vi "Controller Data Server Loop.vi"(4 "Log File Reference":refnum<file>, 7 "Sync Objects":T1, 8 "error in (no error)":errorcluster, 11 "FOFB Configuration":T5={"FOFB Parameters"={"Network"={"FOFB Controller IP"="", "LNLS Control Network IP"="", "LNLS Control Network Power Supplies TCP Port"=0, "LNLS Control Network FOFB Configuration TCP Port"=0, "Data Server TCP Port"=0, "Monitoring Data TCP Port"=0, "Configuration GUI TCP Port"=0, "TCP Listening Timeout"=0}, "Fast Acquisition"={"Acquisition Period"=0, "Data Buffer Size"=0, "Monitoring Period"=0}, "Response Matrix Measurement"={"Step Amplitude"=0.0, "Time Between Steps"=0, "Step Duration"=0, "Number of Averages"=0}, "Correction Algorithm"={"Correction Period"=0, "Reference Orbit Path"=path "", "Response Matrix Path"=path "", "Correction Matrix Path"=path "", "Horizontal Correction Factor"=0.0, "Vertical Correction Factor"=0.0, "Beam Current FOFB Threshold"=0.0, "Decouple H-V"=FALSE, "Use Additional BPM LPF"=FALSE, "BPM LPF Cutoff"=0.0}, "Acquisition Network"=[], "Actuation Network"=[]}, "Number of Acquisition Chassis"=0, "Number of Actuation Chassis"=0, "Number of BPM Readings"=0, "BPM Reading Names"=[], "Selected BPM Readings"=[0, 1, 2, 3, 4, 5, 6, 7, 8, 9, 10, 11, 12, 13, 14, 15, 16, 17, 18, 19, 20, 21, 22, 23, 24, 25, 26, 27, 28, 29, 30, 31, 32, 33, 34, 35, 36, 37, 38, 39, 40, 41, 42, 43, 44, 45, 46, 47, 48, 49], "Number of Correctors"=0, "Corrector Names"=[], "Selected Correctors"=[0, 1, 2, 3, 4, 5, 6, 7, 8, 9, 10, 11, 12, 13, 14, 15, 16, 17, 18, 19, 20, 21, 22, 23, 24, 25, 26, 27, 28, 29, 30, 31, 32, 33, 34, 35, 36, 37, 38, 39, 40, 41, 42, 43, 44, 45, 46, 47, 48, 49], "Reference Orbit"=[], "Response Matrix"=[], "Correction Matrix"=[], "Acquisition Chassis Names"=[], "Actuation Chassis Names"=[], "Acquisition Variables"=[], "Actuation Variables"=[], "PS Matrix Mapping"=[], "Inverse PS Matrix Mapping"=[], "Response Matrix Beam Energy (MeV)"=0.0, "PID Parameters"=[], "BPM Planes"=[], "Corrector Planes"=[], "RMM Step Factor"=[]}) -> (0 "error out":errorcluster)   [LabVIEW 2011, in "Controller VIs.lvlib"]
uses:
  Controller VIs.lvlib
  Types Definitions/Type FOFB Configuration.ctl
  Types Definitions/Type FOFB Parameters.ctl
  Types Definitions/Type Network Configuration.ctl
  Types Definitions/Type FA Configuration.ctl
  Types Definitions/Type Response Matrix Measurement Configuration.ctl
  Types Definitions/Type Correction Algorithm Configuration.ctl
  Types Definitions/Type Acquisition Network Configuration.ctl
  Types Definitions/Type Actuation Network Configuration.ctl
  Types Definitions/Type PID Parameters.ctl
  Types Definitions/Type Synchronization Objects.ctl
  Types Definitions/Type Blocking Synchronization Objects.ctl
  Types Definitions/Type FA Request Parameters.ctl
  Types Definitions/Type BPM and PS select cluster.ctl
  Types Definitions/Type FA File Parameters.ctl
  Types Definitions/Type Monitoring Data.ctl
  Types Definitions/Type Diagnostics Data.ctl
  Types Definitions/Type CPU Loads Array.ctl
  Types Definitions/Type CPU Loads.ctl
  Types Definitions/Type Non-blocking Synchronization Objects.ctl
  Types Definitions/Type FOFB Variables.ctl
  Types Definitions/Type Actuation State.ctl
  <vilib>/Platform/TimedLoop/XDataNode/timing_clust.ctl
  <vilib>/Platform/TimedLoop/XDataNode/nitl_modes.ctl
  <vilib>/Platform/TimedLoop/XDataNode/wakeup.ctl
  <vilib>/rtutility.llb/RT Debug String.vi
  <vilib>/Platform/TimedLoop/XDataNode/XDataNode.xnode
  Data Server VIs.lvlib
  Log VIs.lvlib
  Type Definitions.lvlib
  <vilib>/Platform/TimedLoop/XDataNode/XDNodeRunTimeDep.lvlib
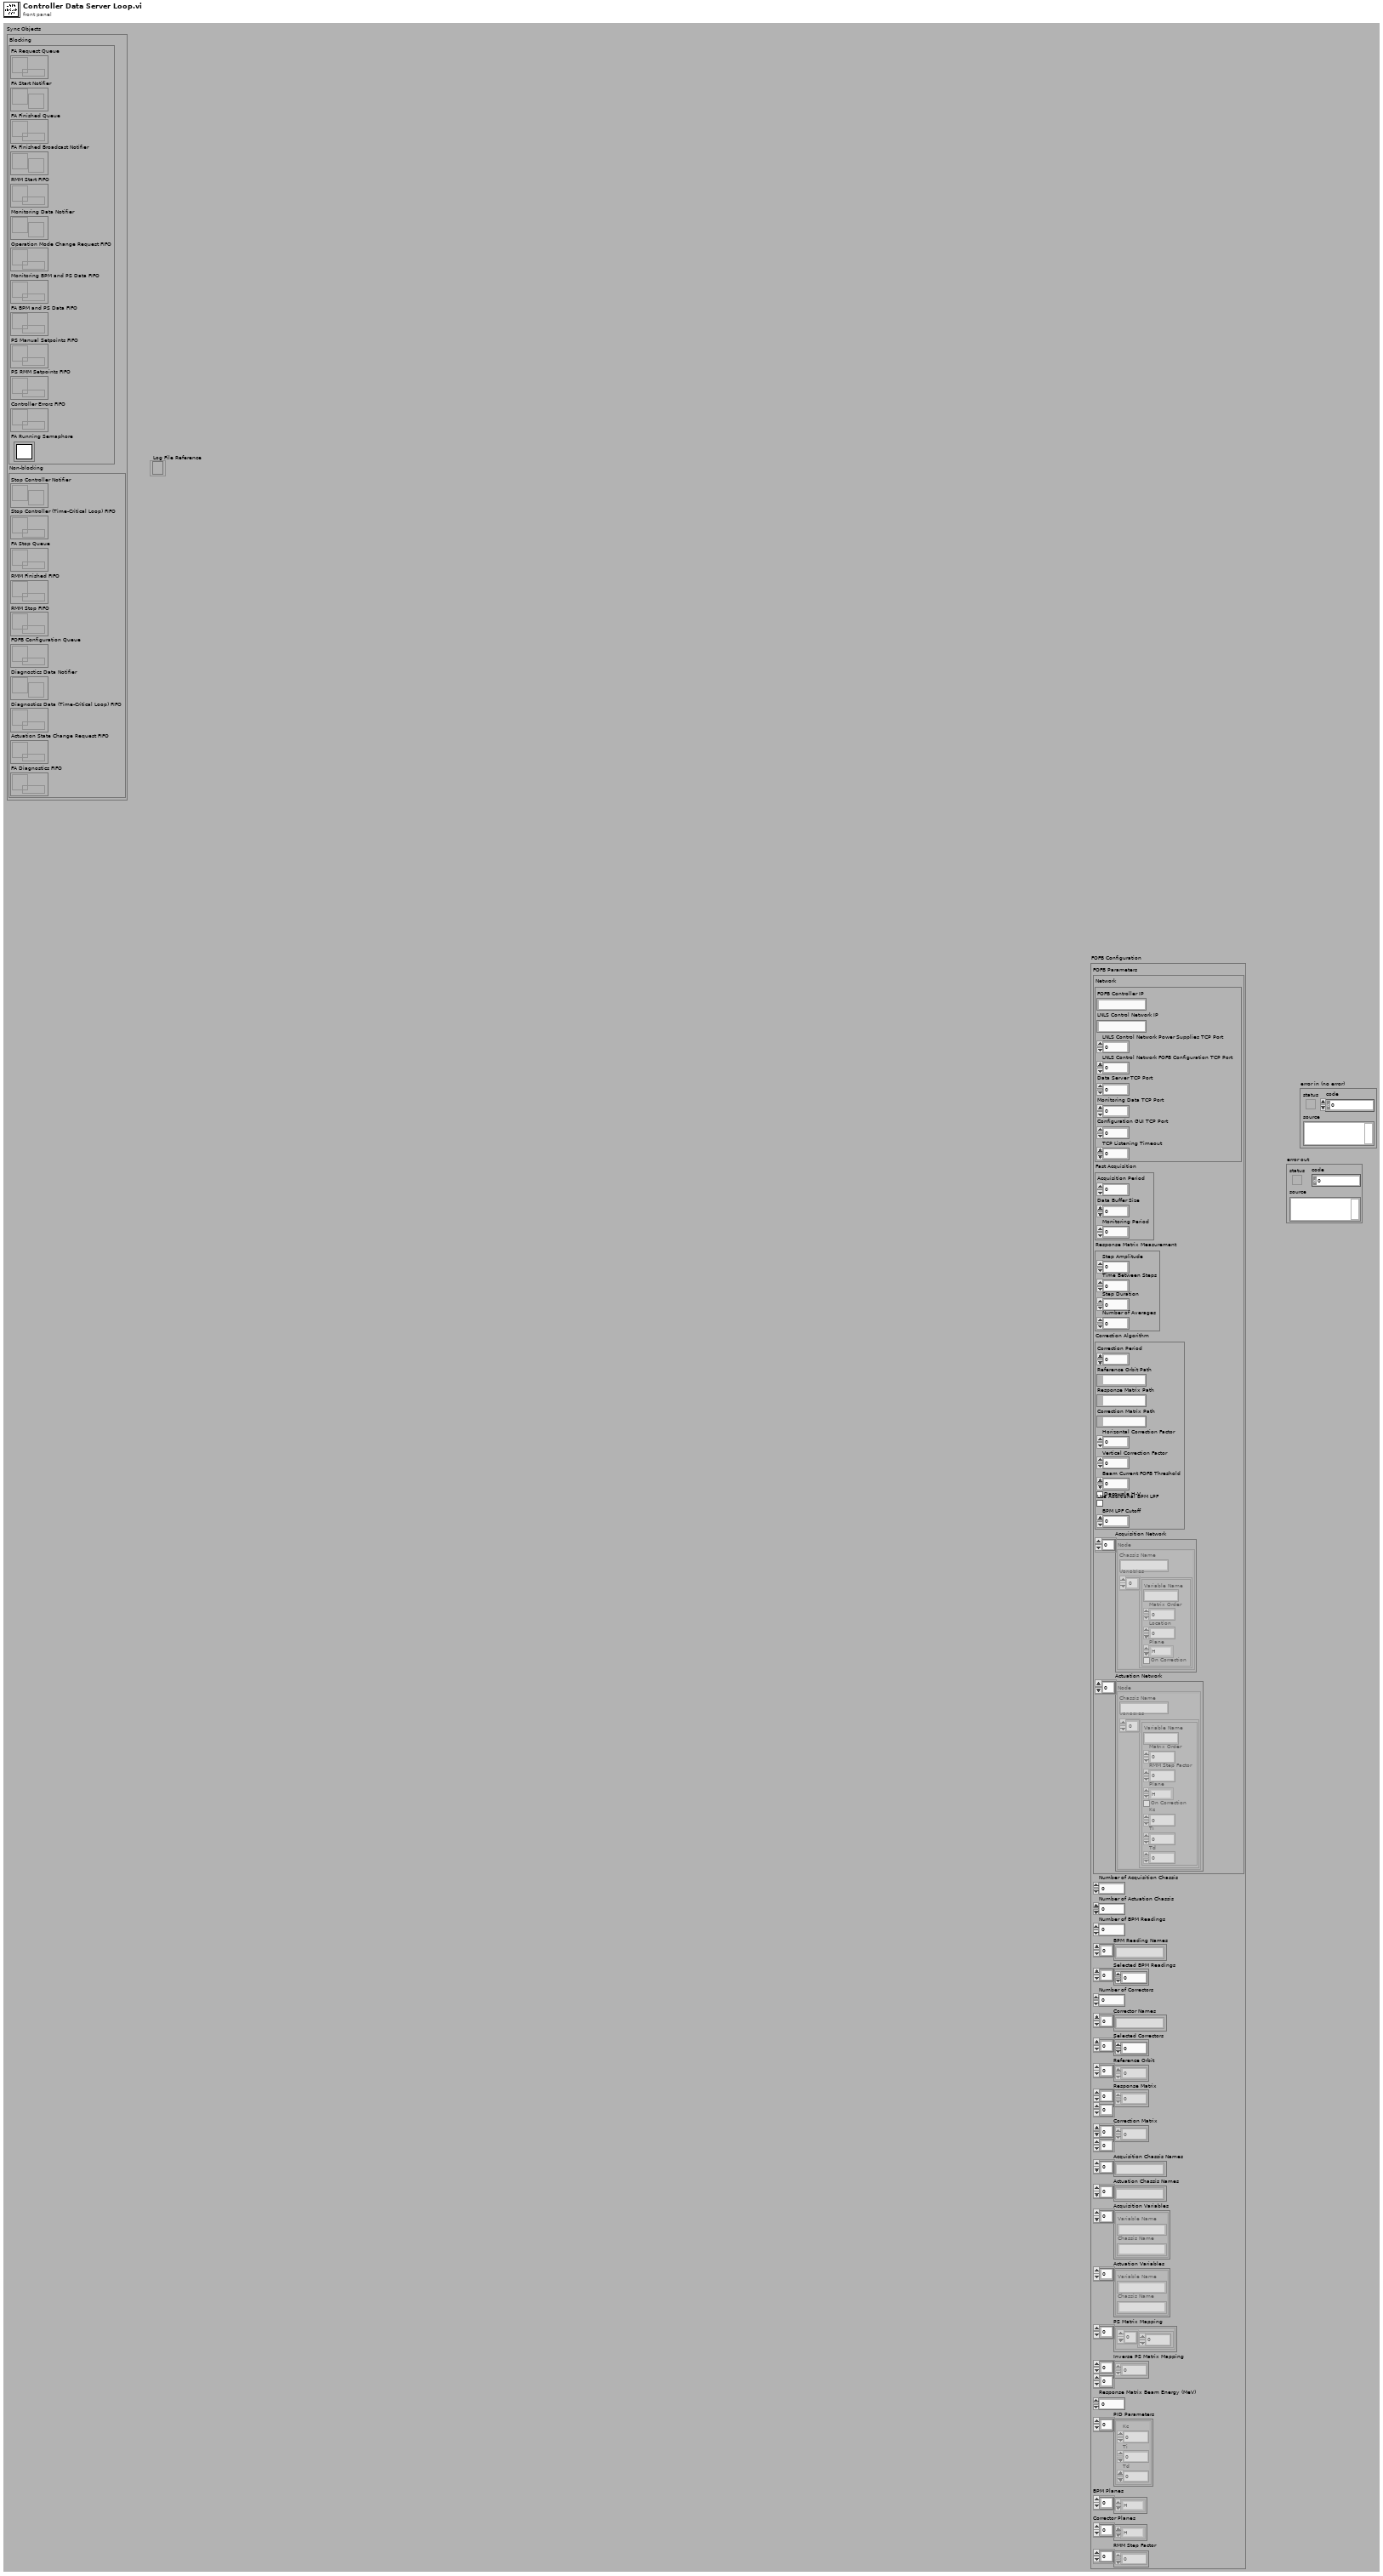
[diagram p1: front panel]
types:
  T1 = typedef "Type Definitions.lvlib/Type Synchronization Objects.ctl" = cluster{"Blocking":T2, "Non-blocking":T4}
  T2 = typedef "Type Definitions.lvlib/Type Blocking Synchronization Objects.ctl" = cluster{"FA Request Queue":refnum<queue>, "FA Start Notifier":refnum<notifier>, "FA Finished Queue":refnum<queue>, "FA Finished Broadcast Notifier":refnum<notifier>, "RMM Start FIFO":refnum<k33>, "Monitoring Data Notifier":refnum<notifier>, "Operation Mode Change Request FIFO":refnum<k33>, "Monitoring BPM and PS Data FIFO":refnum<k33>, "FA BPM and PS Data FIFO":refnum<k33>, "PS Manual Setpoints FIFO":refnum<k33>, "PS RMM Setpoints FIFO":refnum<k33>, "Controller Errors FIFO":refnum<k33>, "FA Running Semaphore":T3}
  T3 = typedef "Semaphore RefNum" = refnum<k1>
  T4 = typedef "Type Definitions.lvlib/Type Non-blocking Synchronization Objects.ctl" = cluster{"Stop Controller Notifier":refnum<notifier>, "Stop Controller (Time-Critical Loop) FIFO":refnum<k33>, "FA Stop Queue":refnum<queue>, "RMM Finished FIFO":refnum<k33>, "RMM Stop FIFO":refnum<k33>, "FOFB Configuration Queue":refnum<queue>, "Diagnostics Data Notifier":refnum<notifier>, "Diagnostics Data (Time-Critical Loop) FIFO":refnum<k33>, "Actuation State Change Request FIFO":refnum<k33>, "FA Diagnostics FIFO":refnum<k33>}
  T5 = typedef "Type Definitions.lvlib/Type FOFB Configuration.ctl" = cluster{"FOFB Parameters":T6, "Number of Acquisition Chassis":i32, "Number of Actuation Chassis":i32, "Number of BPM Readings":i32, "BPM Reading Names":string[], "Selected BPM Readings":u32[], "Number of Correctors":i32, "Corrector Names":string[], "Selected Correctors":u32[], "Reference Orbit":dbl[], "Response Matrix":dbl[][], "Correction Matrix":dbl[][], "Acquisition Chassis Names":string[], "Actuation Chassis Names":string[], "Acquisition Variables":cluster{"Variable Name":string, "Chassis Name":string}[], "Actuation Variables":cluster{"Variable Name":string, "Chassis Name":string}[], "PS Matrix Mapping":cluster{u32[]}[], "Inverse PS Matrix Mapping":u32[][], "Response Matrix Beam Energy (MeV)":dbl, "PID Parameters":T13[], "BPM Planes":enum8{"H", "V"}[], "Corrector Planes":enum8{"H", "V"}[], "RMM Step Factor":dbl[]}
  T6 = typedef "Type Definitions.lvlib/Type FOFB Parameters.ctl" = cluster{"Network":T7, "Fast Acquisition":T8, "Response Matrix Measurement":T9, "Correction Algorithm":T10, "Acquisition Network":T11, "Actuation Network":T12}
  T7 = typedef "Type Definitions.lvlib/Type Network Configuration.ctl" = cluster{"FOFB Controller IP":string, "LNLS Control Network IP":string, "LNLS Control Network Power Supplies TCP Port":u16, "LNLS Control Network FOFB Configuration TCP Port":u16, "Data Server TCP Port":u16, "Monitoring Data TCP Port":u16, "Configuration GUI TCP Port":u16, "TCP Listening Timeout":i32}
  T8 = typedef "Type Definitions.lvlib/Type FA Configuration.ctl" = cluster{"Acquisition Period":u32, "Data Buffer Size":u32, "Monitoring Period":u32}
  T9 = typedef "Type Definitions.lvlib/Type Response Matrix Measurement Configuration.ctl" = cluster{"Step Amplitude":dbl, "Time Between Steps":u32, "Step Duration":u32, "Number of Averages":u32}
  T10 = typedef "Type Definitions.lvlib/Type Correction Algorithm Configuration.ctl" = cluster{"Correction Period":u32, "Reference Orbit Path":path, "Response Matrix Path":path, "Correction Matrix Path":path, "Horizontal Correction Factor":dbl, "Vertical Correction Factor":dbl, "Beam Current FOFB Threshold":dbl, "Decouple H-V":bool, "Use Additional BPM LPF":bool, "BPM LPF Cutoff":dbl}
  T11 = typedef "Type Definitions.lvlib/Type Acquisition Network Configuration.ctl" = cluster{"Chassis Name":string, "Variables":cluster{"Variable Name":string, "Matrix Order":u32, "Location":dbl, "Plane":enum8{"H", "V"}, "On Correction":bool}[]}[]
  T12 = typedef "Type Definitions.lvlib/Type Actuation Network Configuration.ctl" = cluster{"Chassis Name":string, "Variables":cluster{"Variable Name":string, "Matrix Order":u32, "RMM Step Factor":dbl, "Plane":enum8{"H", "V"}, "On Correction":bool, "Kc":dbl, "Ti":dbl, "Td":dbl}[]}[]
  T13 = typedef "Type Definitions.lvlib/Type PID Parameters.ctl" = cluster{"Kc":fxp<+/-,16,8>, "Ti":fxp<+/-,16,8>, "Td":fxp<+/-,16,8>}
  T14 = enum16{"Wait Connection", "Read Data 1", "Write Data", "Read Data 2", "Close Connection", "Idle"}
  T15 = typedef "XDNodeRunTimeDep.lvlib/timing_clust.ctl" = cluster{"Expected End [f-1]":u64, "Actual End [f-1]":u64, "Finished Late? [f-1]":bool, "Expected End [i-1]":u64, "Actual End [i-1]":u64, "Finished Late? [i-1]":bool, "Expected Start [i]":u64, "Actual Start [i]":u64, "Expected Start [f]":u64, "Actual Start [f]":u64, "Source Name":string, "Structure Name":string, "Period":i64, "Deadline":i64, "Offset":i64, "Start":i64, "Priority":i32, "Timeout":i32, "Mode":T16, "Wakeup Reason":T17, "Error":errorcluster, "Source Type":string, "Secondary Source Type":string, "Global End Time":u64, "Global Start Time":u64, "Frame Duration":u64, "Iteration Duration":u64, "Assigned CPU":i32, "I/O Scan Engine Mode":u32}
  T16 = typedef "XDNodeRunTimeDep.lvlib/nitl_modes.ctl" = enum32{"No Change", "Process missed periods, maintain original phase", "Discard missed periods, maintain original phase", "Process missed periods, ignore original phase", "Discard missed periods, ignore original phase"}
  T17 = typedef "XDNodeRunTimeDep.lvlib/wakeup.ctl" = enum32{"Normal", "Aborted", "Asynchronous wakeup", "Timing source error", "Timed loop error", "Timeout"}
  T18 = enum16{"Standard", "Buffered", "CRLF", "Immediate"}
  T19 = typedef "Type Definitions.lvlib/Type FA Request Parameters.ctl" = cluster{"Number of Samples":u32, "BPM and PS Selection":T20, "Filename":string}
  T20 = typedef "Type Definitions.lvlib/Type BPM and PS select cluster.ctl" = cluster{"BPM index array":u32[], "PS index array ":u32[]}
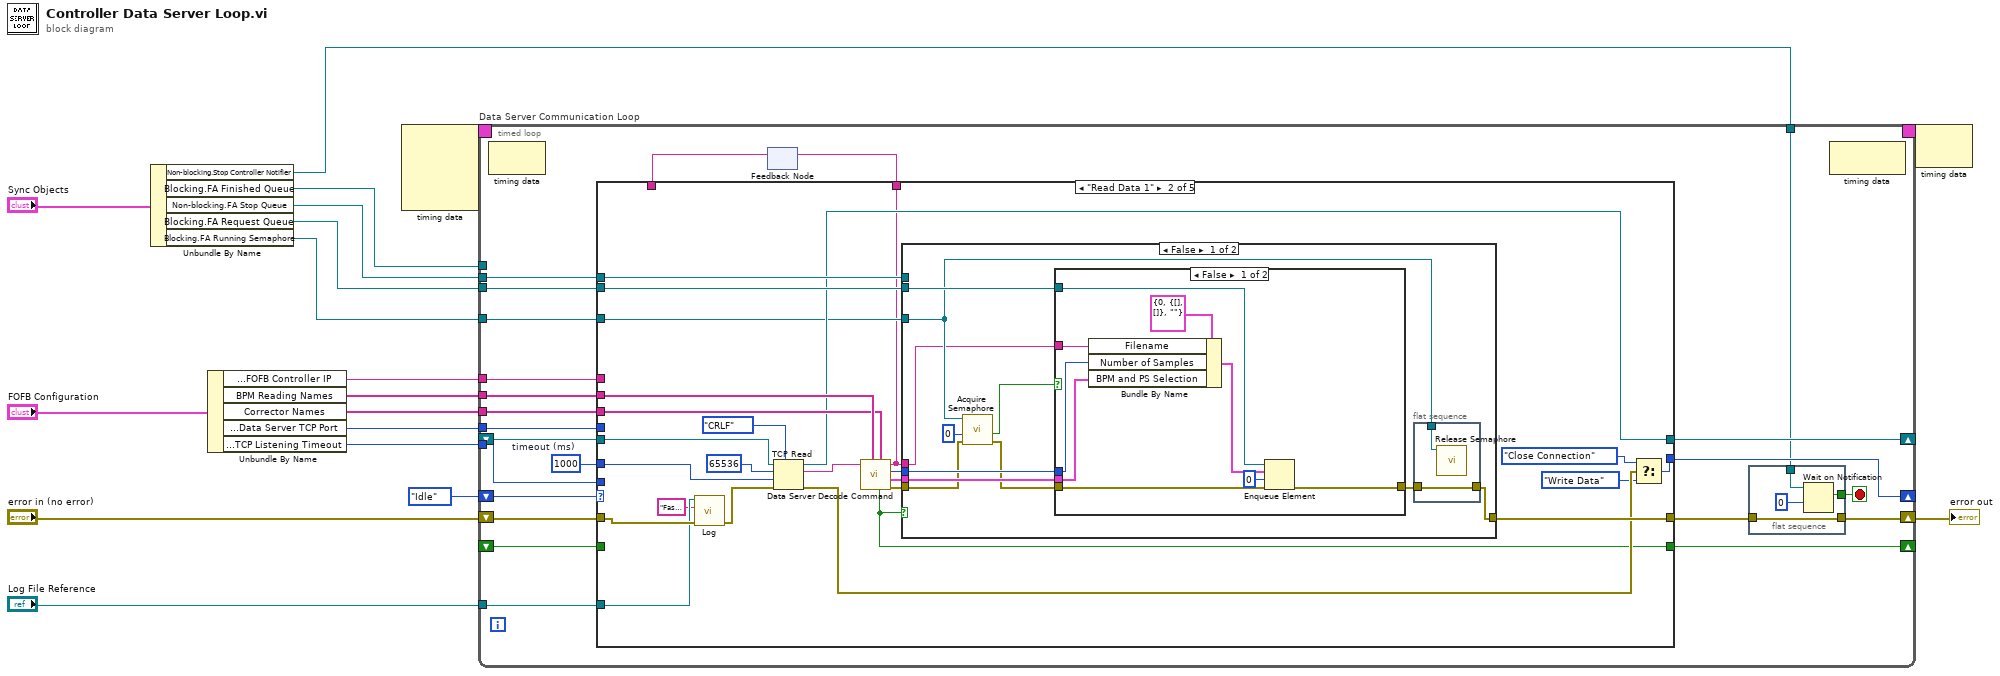
[diagram p0: block diagram]
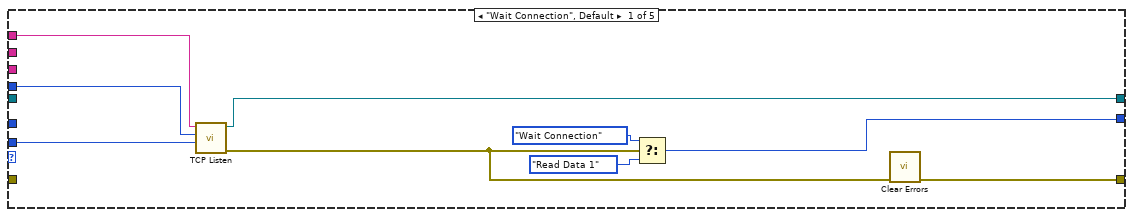
[diagram p2: hidden frame]
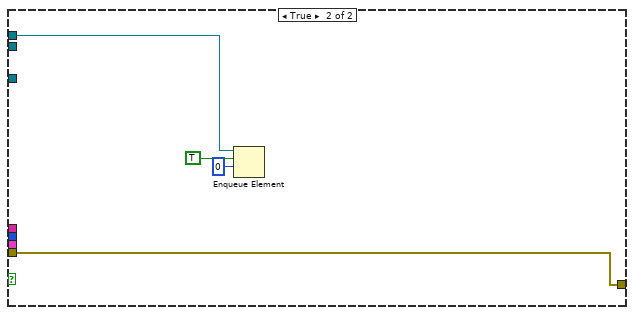
[diagram p4: hidden frame]
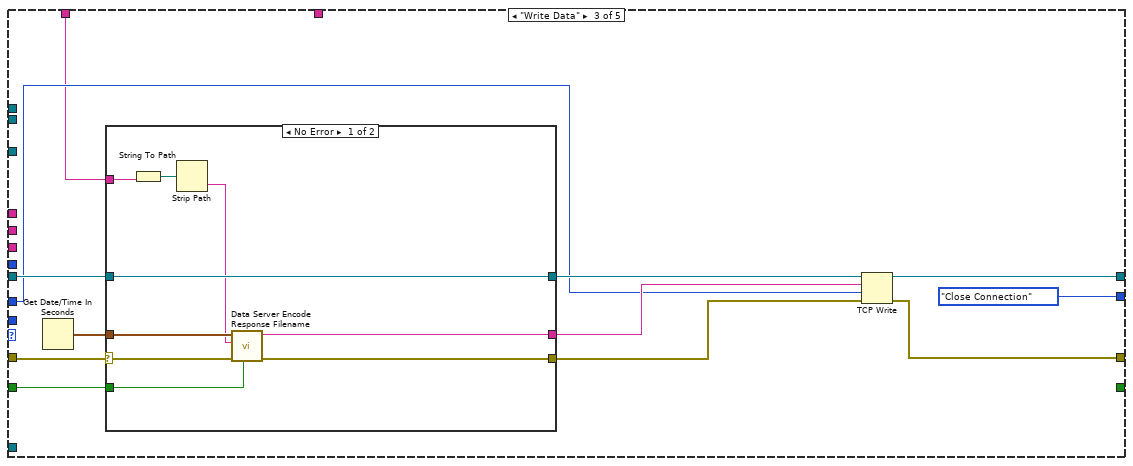
[diagram p5: hidden frame]
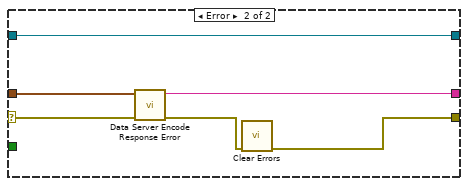
[diagram p6: hidden frame]
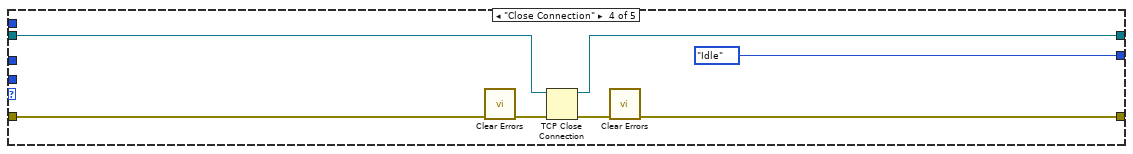
[diagram p7: hidden frame]
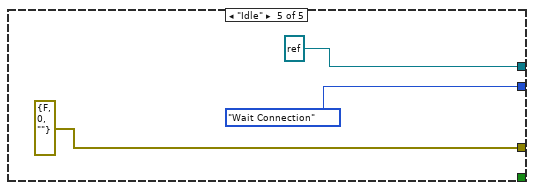
[diagram p8: hidden frame]
diagram:
  n1 = Unbundle By Name("Sync Objects") -> ("Non-blocking.Stop Controller Notifier"=w8:refnum<notifier>, "Blocking.FA Finished Queue"=w4:refnum<queue>, "Non-blocking.FA Stop Queue"=w6:refnum<queue>, "Blocking.FA Request Queue"=w7:refnum<queue>, "Blocking.FA Running Semaphore"=w3:T3)
  n2 = Unbundle By Name("FOFB Configuration") -> ("FOFB Parameters.Network.FOFB Controller IP"=w11:string, "BPM Reading Names"=w12:string[], "Corrector Names"=w13:string[], "FOFB Parameters.Network.Data Server TCP Port"=w9:u16, "FOFB Parameters.Network.TCP Listening Timeout"=w5:i32)
  n3 = node-c288() -> (w2:T15)  [unwired: 4 in]
  n4 = timed-loop "Data Server Communication Loop" {
    shift-right: [w40] -> _
    shift-left: _ -> [w37]
    shift-right: [w39] -> _
    shift-left: T14."Idle" ("f") -> [w41]
    shift-right: [w27] -> w15
    shift-left: "error in (no error)" -> [w38]
    tunnel: w12 -> [w35]
    tunnel: w13 -> [w34]
    tunnel: w11 -> [w33]
    tunnel: w9 -> [w31]
    tunnel: w8 -> [w30]
    tunnel: "Log File Reference" -> [w29]
    tunnel: w7 -> [w26]
    tunnel: w6 -> [w25]
    tunnel: w5 -> [w24]
    shift-right: [w23] -> _
    shift-left: _ -> [w22]
    tunnel: w4 -> [_]
    tunnel: w3 -> [w21]
    timing: w2 -> [_]
    timing-out: [_] -> w1
    stop <- w32 stop-if-true
    w36 = 1000  # timeout (ms)
    # "ms"
    n5 = node-c288() -> ()  [unwired: 1 in, 1 out]
    n6 = feedback #1() -> (w20:string)  [unwired: 1 in]
    n7 = case shown="\"Read Data 1\"" w41 {
      tunnel: [w56 w59 w115 w140 refnum<k5> refnum ("connection ID")] -> w40
      tunnel: [w53 w65 T14."Close Connection" ("f") T14."Idle" ("f") T14."Wait Connection" ("f")] -> w39
      tunnel: [w49 w66 w111 w139 errorcluster {"status"=FALSE, "code"=0, "source"=""} ("error out")] -> w28
      tunnel: w38 -> [_ w74 w120 w136 _]
      tunnel: w37 -> [_ w79 w118 w141 _]
      tunnel: w36 -> [_ w78 w113 _ _]
      tunnel: w35 -> [_ w76 _ _ _]
      tunnel: w34 -> [_ w75 _ _ _]
      tunnel: w33 -> [w52 _ _ _ _]
      tunnel: w31 -> [w51 _ _ _ _]
      tunnel: w29 -> [_ w72 _ _ _]
      tunnel: w26 -> [_ w70 _ _ _]
      tunnel: w25 -> [_ w61 _ _ _]
      tunnel: w24 -> [w48 _ _ _ _]
      tunnel: w22 -> [_ _ w110 _ _]
      tunnel: [_ w60 _ _ _] -> w23
      tunnel: w21 -> [_ w58 _ _ _]
      tunnel: w20 -> [_ _ w109 _ _]
      tunnel: [_ w57 _ _ _] -> w19
      frame "Wait Connection", Default {
        n8 = call <vilib>:"TCP Listen.vi"("timeout ms (wait forever: -1)"=w48, "port"=w51, "service name"=w52) -> ("error out"=w50:errorcluster, "connection ID"=w56:refnum<k5>)  [unwired: 4 in, 3 out]
        n9 = Select(t=T14."Wait Connection" ("f"), s=w50, f=T14."Read Data 1") -> (s? t:f=w53:T14)
        n10 = call <vilib>:"Clear Errors.vi"("error in (no error)"=w50) -> ("error out"=w49:errorcluster)  [unwired: 6 out]
      }
      frame "Read Data 1" {
        n11 = call "Log.vi"("error in (no error)"=w74, "String"="Fast Acquisition requested by user.", "Log File Reference"=w72) -> ("error out"=w73:errorcluster)  [unwired: 7 in, 1 out]
        n12 = TCP Read(connection ID=w79, bytes to read=65536, error in (no error)=w73, 7:T18."CRLF" ("mode (standard)"), 9:w78) -> (connection ID out=w59:refnum<k5>, data out=w77:string, error out=w63:errorcluster)
        n13 = call "Data Server Decode Command.vi"("Corrector names"=w75, "BPM names"=w76, "Input string"=w77) -> ("error out"=w67:errorcluster, "BPM and PS index"=w68:T20, "Number of samples"=w69:u32, "Filename"=w57:string, "Stop Acquisition?"=w60:bool)  [unwired: 4 in]
        n14 = case shown="False" w60 {
          tunnel: w70 -> [w92 _]
          tunnel: w69 -> [w91 _]
          tunnel: w68 -> [w90 _]
          tunnel: w67 -> [w88 w108]
          tunnel: [w83 w108] -> w66
          tunnel: w61 -> [_ w107]
          tunnel: w58 -> [w85 _]
          tunnel: w57 -> [w82 _]
          frame False {
            n15 = call <vilib>:"Acquire Semaphore.vi"("error in (no error)"=w88, "ms timeout (-1)"=0, "semaphore"=w85) -> ("error out"=w87:errorcluster, "timed out"=w86:bool)  [unwired: 2 in, 1 out]
            n16 = case shown="False" w86 {
              tunnel: w92 -> [w99 _]
              tunnel: w91 -> [w102 _]
              tunnel: w90 -> [w101 _]
              tunnel: w82 -> [w100 _]
              tunnel: [w95 w104] -> w84
              tunnel: w87 -> [w97 w104]
              frame False {
                n17 = Bundle By Name(cluster=T19 {"Number of Samples"=0, "BPM and PS Selection"={"BPM index array"=[], "PS index array "=[]}, "Filename"=""} ("notification"), "Filename"=w100, "Number of Samples"=w102, "BPM and PS Selection"=w101) -> (w98:T19)
                n18 = Enqueue Element(queue=w99, element=w98, timeout in ms (-1)=0, error in (no error)=w97) -> (error out=w95:errorcluster)  [unwired: 2 out]
              }
              frame True {
              }
            }
            n19 = flat-sequence {
              tunnel: w85 -> [w94]
              tunnel: w84 -> [w93]
              tunnel: [w93] -> w83
              frame #0 {
                n20 = call <vilib>:"Release Semaphore.vi"("semaphore"=w94) -> ()  [unwired: 5 in, 2 out]
              }
            }
          }
          frame True {
            n21 = Enqueue Element(queue=w107, element=TRUE ("notification"), timeout in ms (-1)=0) -> ()  [unwired: 1 in, 3 out]
          }
        }
        n22 = Select(t=T14."Close Connection" ("f"), s=w63, f=T14."Write Data") -> (s? t:f=w65:T14)
      }
      frame "Write Data" {
        n23 = Get Date/Time In Seconds() -> (seconds since 1Jan1904=w119:timestamp)
        n24 = case shown="No Error" w120 {
          selector: w120 -> [w128 w135]
          tunnel: w119 -> [w129 w134]
          tunnel: [w125 w130] -> w116
          tunnel: w118 -> [w127 w133]
          tunnel: [w127 w133] -> w117
          tunnel: [w126 w131] -> w114
          tunnel: w109 -> [w124 _]
          tunnel: w110 -> [w121 _]
          frame No Error {
            n25 = String To Path(string=w124) -> (path=w123:path)
            n26 = Strip Path(path=w123) -> (name=w122:string)  [unwired: 1 out]
            n27 = call "Data Server Encode Response Filename.vi"("FA Stopped?"=w121, "error in (no error)"=w128, "Filename"=w122, "Time Stamp"=w129) -> ("error out"=w126:errorcluster, "Output string"=w125:string)  [unwired: 6 in]
          }
          frame Error {
            n28 = call "Data Server Encode Response Error.vi"("error in (no error)"=w135, "Time Stamp"=w134) -> ("error out"=w132:errorcluster, "Output string"=w130:string)  [unwired: 8 in]
            n29 = call <vilib>:"Clear Errors.vi"("error in (no error)"=w132) -> ("error out"=w131:errorcluster)  [unwired: 6 in]
          }
        }
        n30 = TCP Write(connection ID=w117, data in=w116, error in (no error)=w114, 9:w113) -> (connection ID out=w115:refnum<k5>, error out=w111:errorcluster)  [unwired: 1 out]
      }
      frame "Close Connection" {
        n31 = call <vilib>:"Clear Errors.vi"("error in (no error)"=w136) -> ("error out"=w138:errorcluster)  [unwired: 6 in]
        n32 = TCP Close Connection(connection ID=w141, error in (no error)=w138) -> (connection ID out=w140:refnum<k5>, error out=w137:errorcluster)  [unwired: 1 in]
        n33 = call <vilib>:"Clear Errors.vi"("error in (no error)"=w137) -> ("error out"=w139:errorcluster)  [unwired: 6 in]
      }
      frame "Idle" {
      }
    }
    n34 = feedback-in #1(w19) -> ()
    n35 = flat-sequence {
      tunnel: [w46] -> w32
      tunnel: w30 -> [w45]
      tunnel: w28 -> [w44]
      tunnel: [w44] -> w27
      frame #0 {
        n36 = Wait on Notification(notifier=w45, timeout in ms (-1)=0) -> (notification=w46:bool)  [unwired: 2 in, 3 out]
      }
    }
    n37 = node-c288() -> ()  [unwired: 1 in, 1 out]
  }
  "error out" <- w15
  n38 = node-c288(w1) -> ()  [unwired: 1 out]
